vi "visa读取串口字节(1).vi"() -> ()   [LabVIEW 2012]
uses:
  <vilib>/Instr/_visa.llb/VISA Configure Serial Port (Instr).vi
panel:
  out "读取缓冲区":string
  in  "停止":bool
  in  "启用终止符":bool
  in  "flow control":u16(ring) caption="流程控制" items=["无"=0, "XON/XOFF"=1, "RTS/CTS"=2, "DTR/DSR"=4]
  in  "stop bits":u16(ring)=10 caption="停止位" items=["1.0"=10, "1.5"=15, "2.0"=20]
  in  "parity":u16(ring) caption="奇偶" items=["无", "奇", "偶", "标记", "空格"]
  in  "data bits":u16=8 caption="数据比特" min=5 max=8 step=1
  in  "VISA resource name":refnum<visa-resource-name>="COM1" caption="VISA资源名称"
  in  "baud rate":u32=9600 caption="波特率"
  # "简单的读取串口字节"
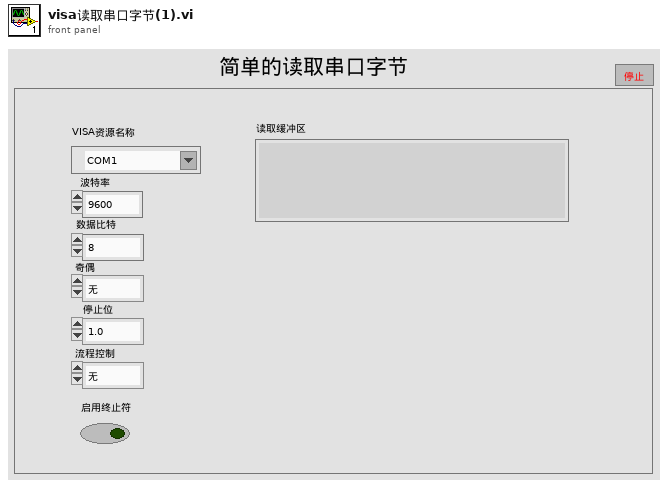
[diagram p1: front panel]
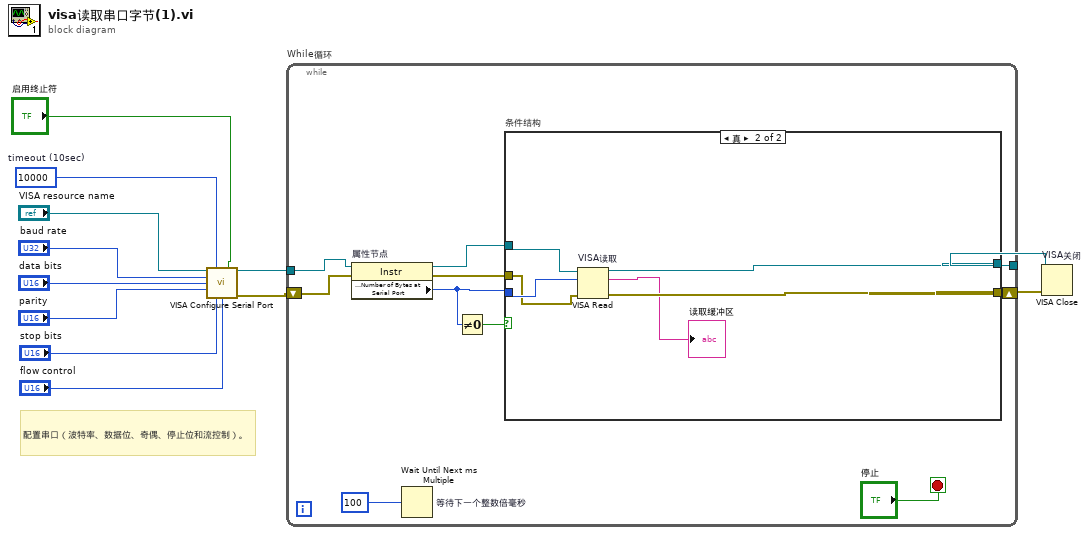
[diagram p0: block diagram]
diagram:
  w9 = u32 10000  # timeout (10sec)
  # "配置串口（波特率、数据位、奇偶、停止位和流控制）。"
  n1 = call-poly "VISA Configure Serial Port"("VISA resource name"="VISA resource name", "timeout (10sec)"=w9, "Enable Termination\nChar (T)"="启用终止符", "baud rate (9600)"="baud rate", "data bits (8)"="data bits", "parity (0:none)"="parity", "stop bits (10: 1 bit)"="stop bits", "flow control (0:none)"="flow control") -> ("VISA resource name out"=w2:refnum<visa-resource-name>, "error out"=w4:errorcluster)  [unwired: 1 in, 5 out]
  n2 = while "While循环" {
    shift-right: [w15] -> w3
    shift-left: w4 -> [w21]
    tunnel: w2 -> [w20]
    tunnel: [w14] -> w1
    stop <- "停止" stop-if-true
    n3 = property on="属性节点" class="Instr"(reference=w20, error in=w21) -> (reference out=w16:refnum<visa-resource-name>, error out=w13:errorcluster, "Serial Settings:Number of Bytes at Serial Port"=w17:u32)
    n4 = Wait Until Next ms Multiple "等待下一个整数倍毫秒"(millisecond multiple=u32 100 ("毫秒倍数")) -> ()  [unwired: 1 out]
    n5 = Not Equal To 0?(x=w17) -> (x != 0?=w18:bool)
    n6 = case "条件结构" shown="真" w18 {
      tunnel: w17 -> [_ w30]
      tunnel: w16 -> [w24 w29]
      tunnel: [w23 w28] -> w15
      tunnel: [w24 w27] -> w14
      tunnel: w13 -> [w23 w26]
      frame False {
      }
      frame True {
        n7 = VISA Read "VISA读取"(VISA resource name=w29, byte count=w30, error in (no error)=w26) -> (VISA resource name out=w27:refnum<visa-resource-name>, read buffer=→"读取缓冲区":string, error out=w28:errorcluster)  [unwired: 1 out]
      }
    }
  }
  n8 = VISA Close "VISA关闭"(VISA resource name=w1, error in (no error)=w3) -> ()  [unwired: 1 out]
